vi "send all action command.vi"(8 "error in":errorcluster, 10 "commands":T1, 11 "message queue in":T2) -> (0 "error out":errorcluster, 3 "message queue out":T2)   [LabVIEW 2013, in "module execution process.lvlib"]
doc: "Use this VI to send any commands that don't require additional inputs. It is essentially a catch-all for all the commands that don't already have their own VI."
uses:
  module execution process.lvlib
  <vilib>/NI/AMC/Message Queue.ctl
  <vilib>/NI/AMC/Message.ctl
  <vilib>/NI/Tools/Keyed Array/KeyedArray.ctl
  command commands to rtexe process.ctl
  <vilib>/NI/AMC/Create Single Message.vi
  <vilib>/NI/AMC/Update Message Routing Info.vi
  <vilib>/NI/AMC/Send Message.vi
  <vilib>/NI/AMC/AMC.lvlib
  <vilib>/NI/Tools/Keyed Array/Tools_KeyedArray.lvlib
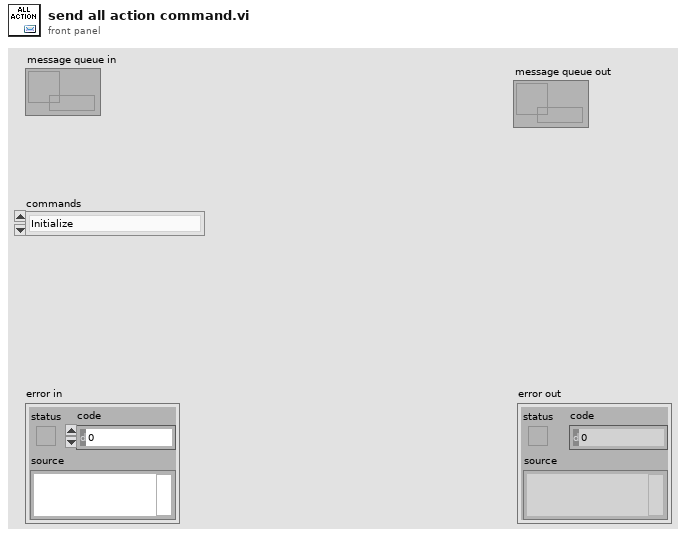
[diagram p1: front panel]
types:
  T1 = typedef "module execution process.lvlib/command commands to rtexe process.ctl" = enum16{"Initialize", "Add Search Paths", "Load from File", "Unload File", "Open All Engines", "Open Single Engine", "Initialize All Engines", "Initialize Single Engine", "Start All", "Start Single", "Pause All", "Pause Single", "Stop All", "Stop Single", "Close All", "Close Single", "Set Safe State All", "Set Safe State Single", "Get Status", "Exit", "Error", "Load Bitfile", "Unload Bitfile", "Clear Faults Single", "Clear Faults All"}
  T2 = typedef "AMC.lvlib/Message Queue.ctl" = refnum<queue>
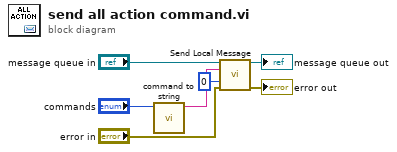
[diagram p0: block diagram]
diagram:
  n1 = call "command to string.vi"("commands"="commands") -> ("command string"=w3:string)  [unwired: 10 in]
  n2 = call <vilib>:"Send Local Message.vi"("message queue in"="message queue in", "message name"=w3, "timeout (-1 ms)"=0, "error in"="error in") -> ("message queue out"=→"message queue out":T2, "error out"=→"error out":errorcluster)  [unwired: 9 in, 1 out]
